vi "Theme5_Topic1_qn6.vi"(9 "RefPrevious":refnum<vi>, 10 "RefNext":refnum<vi>, 11 "connection reference":T1) -> (2 "AnsIndicator":refnum<vi>[](array[refnum]))   [LabVIEW 2013]
uses:
  why.vi
  Precontrol.vi
  <vilib>/addons/database/Connection.llb/Conn ObjectReference.ctl
  <vilib>/addons/database/NI_Database_API.lvlib
panel:
  out "Why?":string
  out "DInd":bool
  out "CInd":bool
  out "BInd":bool
  out "AInd":bool
  in  "ABCD":enum32{"No Selection", "A", "B", "C", "D"}(radio)
  out "MCQ_Randomized":string[](array[string])
  # "What happens when a positive test charge is brought in the vicinity of another positive\ntest charge?"
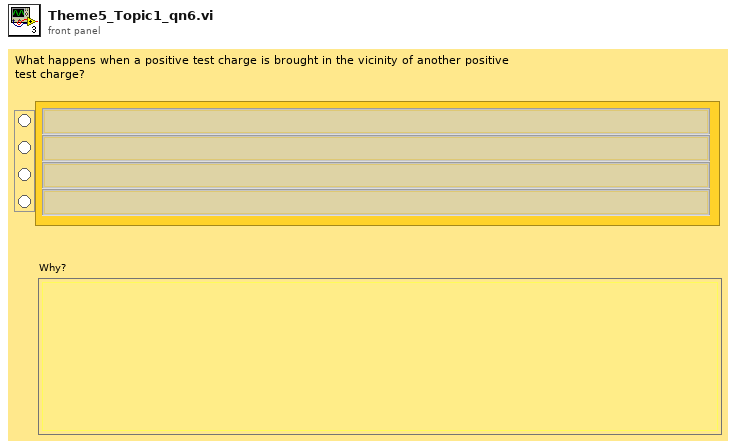
[diagram p1: front panel]
types:
  T1 = typedef "NI_Database_API.lvlib/Conn ObjectReference.ctl" = refnum<k1>
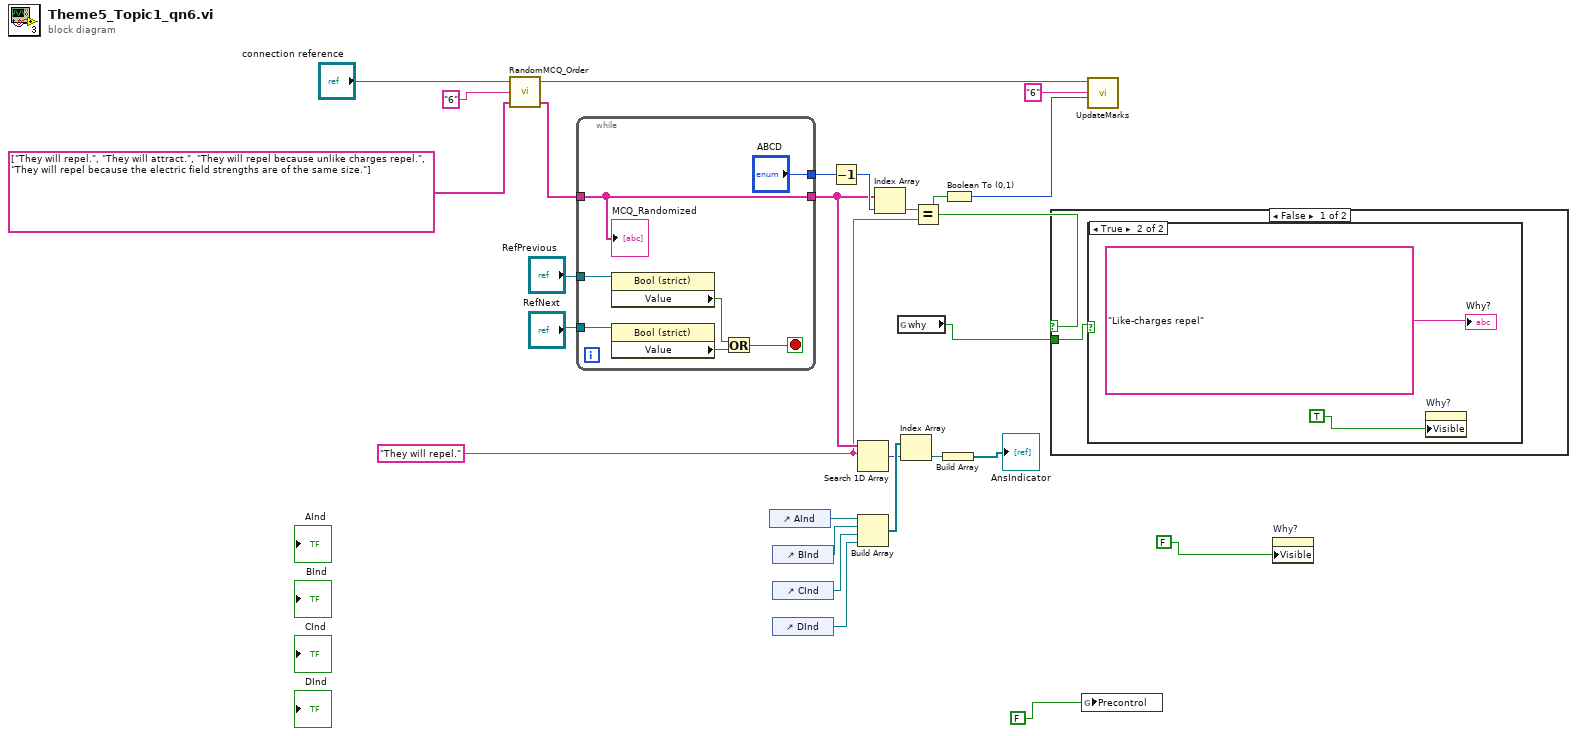
[diagram p0: block diagram]
diagram:
  w12 = "They will repel." ("element")
  n1 = call "RandomMCQ_Order.vi"("MCQ_Ordered"=string[] ["They will repel.", "They will attract.", "They will repel because unlike charges repel.", "They will repel because the electric field strengths are of the same size."], "Questions_Ordered"="6", "connection reference"="connection reference") -> ("MCQ_Randomized"=w26:string[], "connection reference out"=w9:T1)  [unwired: 1 in]
  n2 = while {
    tunnel: ["ABCD"] -> w16
    tunnel: w26 -> [w28]
    tunnel: [w28] -> w14
    tunnel: "RefNext" -> [w29]
    tunnel: "RefPrevious" -> [w30]
    stop <- w27 stop-if-true
    n3 = property class="Bool (strict)"(reference=w30) -> ("Value"=w32:bool)  [unwired: 1 in, 2 out]
    n4 = property class="Bool (strict)"(reference=w29) -> ("Value"=w31:bool)  [unwired: 1 in, 2 out]
    n5 = Or(x=w32, y=w31) -> (x .or. y?=w27:bool)
    "MCQ_Randomized" <- w28
  }
  n6 = control-ref of="AInd"() -> (w23:refnum<vi>)
  n7 = control-ref of="BInd"() -> (w22:refnum<vi>)
  n8 = control-ref of="CInd"() -> (w21:refnum<vi>)
  n9 = control-ref of="DInd"() -> (w20:refnum<vi>)
  n10 = Decrement(x=w16) -> (x-1=w15:enum32{"No Selection", "A", "B", "C", "D"})
  n11 = Search 1D Array(1D array=w14, element=w12) -> (index of element=w18:i32)  [unwired: 1 in]
  n12 = Build Array(w23, w22, w21, w20) -> (w19:refnum<vi>[])
  n13 = Index Array(array=w14, index=w15) -> (element=w13:string)
  n14 = global read "why.vi" "why"() -> (w2:bool)
  n15 = Index Array(array=w19, index=w18) -> (element=w17:refnum<vi>)
  n16 = Equal?(x=w13, y=w12) -> (x = y?=w4:bool)
  n17 = Build Array(w17) -> (→"AnsIndicator":refnum<vi>[])
  n18 = Boolean To (0,1)(Boolean=w4) -> (0, 1=w5:i16)
  n19 = case shown="False" w4 {
    tunnel: w2 -> [w34 _]
    frame False {
      n20 = case shown="True" w34 {
        frame False {
        }
        frame True {
          n21 = property on="Why?" class="Str"("Visible"=TRUE) -> ()  [unwired: 2 in, 2 out]
          "Why?" <- "Like-charges repel"
        }
      }
    }
    frame True {
    }
  }
  n22 = global write "Precontrol.vi" "Precontrol"(FALSE) -> ()
  n23 = call "UpdateMarks.vi"("MarksEarned"=w5, "QuestionsNo_Ordered"="6", "connection reference"=w9) -> ()  [unwired: 9 in]
  n24 = property on="Why?" class="Str"("Visible"=FALSE) -> ()  [unwired: 2 in, 2 out]
